vi "camera-get-info-subvi.vi"() -> (0 "error out":errorcluster, 3 "Camera Properties":T1)   [LabVIEW 2014]
uses:
  lib/Andorlib/atmcd32d.lvlib
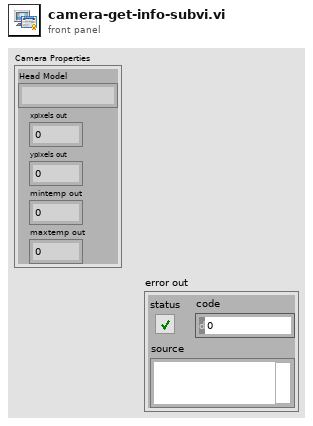
[diagram p1: front panel]
types:
  T1 = cluster{"Head Model":string, "xpixels out":i32, "ypixels out":i32, "mintemp out":i32, "maxtemp out":i32}
  T2 = cluster{"name out":string, "xpixels out":i32, "ypixels out":i32, "mintemp out":i32, "maxtemp out":i32}
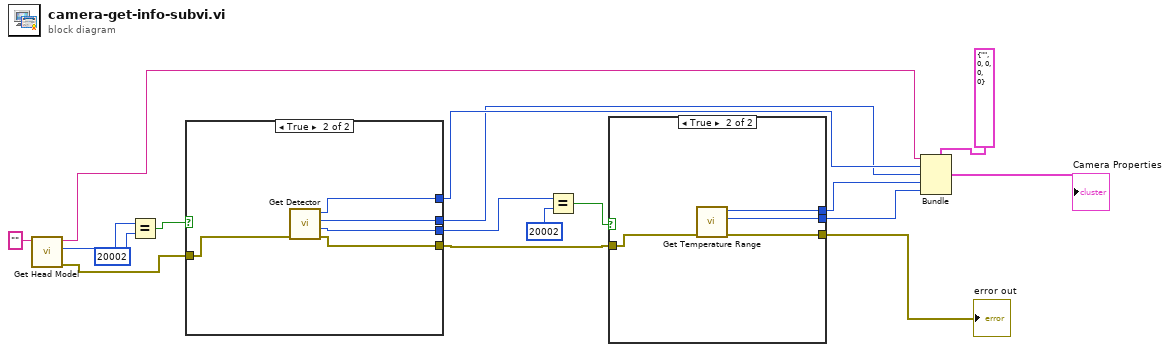
[diagram p0: block diagram]
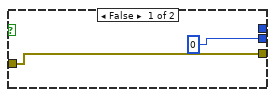
[diagram p3: hidden frame]
diagram:
  n1 = call "Get Head Model.vi"("name"="") -> ("error out"=w13:errorcluster, "function return"=w16:u32, "name out"=w8:string)  [unwired: 8 in]
  n2 = Equal?(x=w16, y=u32 20002) -> (x = y?=w14:bool)
  n3 = case shown="True" w14 {
    tunnel: w13 -> [w19 w24]
    tunnel: [_ w23] -> w6
    tunnel: [_ w22] -> w7
    tunnel: [w19 w21] -> w9
    tunnel: [0 w20] -> w11
    frame False {
    }
    frame True {
      n4 = call "Get Detector.vi"("error in (no error)"=w24) -> ("error out"=w21:errorcluster, "function return"=w20:u32, "ypixels out"=w23:i32, "xpixels out"=w22:i32)  [unwired: 7 in]
    }
  }
  n5 = Equal?(x=w11, y=u32 20002) -> (x = y?=w10:bool)
  n6 = case shown="True" w10 {
    tunnel: w9 -> [w25 w29]
    tunnel: [_ w28] -> w5
    tunnel: [_ w27] -> w4
    tunnel: [w25 w26] -> w1
    frame False {
    }
    frame True {
      n7 = call "Get Temperature Range.vi"("error in (no error)"=w29) -> ("error out"=w26:errorcluster, "maxtemp out"=w27:i32, "mintemp out"=w28:i32)  [unwired: 7 in, 1 out]
    }
  }
  "error out" <- w1
  n8 = Bundle(cluster=T2 {"name out"="", "xpixels out"=0, "ypixels out"=0, "mintemp out"=0, "maxtemp out"=0}, "name out"=w8, "xpixels out"=w7, "ypixels out"=w6, "mintemp out"=w5, "maxtemp out"=w4) -> (→"Camera Properties":T2)
